vi "Enter into hierarchy.vi"(8 "error in (no error)":errorcluster, 10 "output array of keys":string[](array[string]), 11 "Variant in":variant) -> (0 "error out":errorcluster, 3 "Variant out":variant)   [LabVIEW 2015]
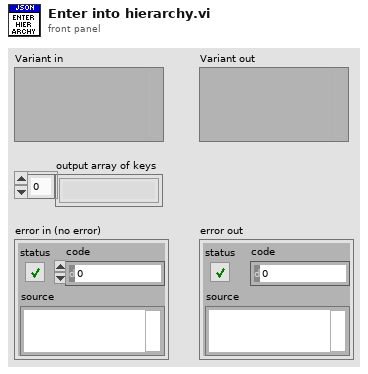
[diagram p1: front panel]
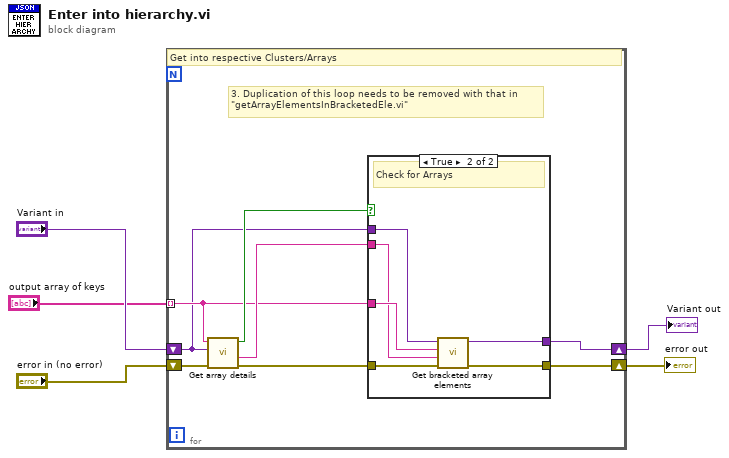
[diagram p0: block diagram]
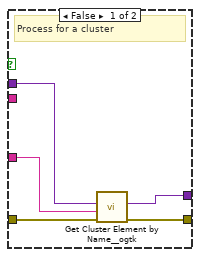
[diagram p2: hidden frame]
diagram:
  n1 = for {
    tunnel: "output array of keys" -> [w8] mode=indexing
    shift-right: [w6] -> w4
    shift-left: "Variant in" -> [w7]
    shift-right: [w13] -> w5
    shift-left: "error in (no error)" -> [w12]
    # "3. Duplication of this loop needs to be removed with that in \n\"getArrayElementsInBracketedEle.vi\""
    # "Get into respective Clusters/Arrays"
    n2 = call "Get array details.vi"("error in (no error)"=w12, "Current obejct"=w7, "Separate object string"=w8) -> ("error out"=w11:errorcluster, "Required object"=w10:string, "Is array?"=w9:bool)  [unwired: 3 in, 3 out]
    n3 = case shown="True" w9 {
      tunnel: w8 -> [w14 w23]
      tunnel: w7 -> [w18 w20]
      tunnel: [w17 w19] -> w6
      tunnel: w11 -> [w16 w24]
      tunnel: [w15 w21] -> w13
      tunnel: w10 -> [_ w22]
      frame False {
        # "Process for a cluster"
        n4 = call <userlib>:"Get Cluster Element by Name__ogtk.vi"("error in (no error)"=w16, "Element Name"=w14, "Cluster"=w18) -> ("error out"=w15:errorcluster, "VElement"=w17:variant)  [unwired: 6 in, 1 out]
      }
      frame True {
        # "Check for Arrays"
        n5 = call "Get bracketed array elements.vi"("error in (no error)"=w24, "requriedObject"=w22, "brackettedElements"=w23, "Variant in"=w20) -> ("error out"=w21:errorcluster, "Array Element"=w19:variant)  [unwired: 5 in, 1 out]
      }
    }
  }
  "error out" <- w5
  "Variant out" <- w4
